vi "Update Step Descriptions.vi"(7 "Action":T1, 10 "Mouse Interaction Tag":string, 11 "UI Data in":refnum<class "Settings UI.lvclass">) -> (3 "UI Data out":refnum<class "Settings UI.lvclass">)   [LabVIEW 2020, in "Output Sequencer.lvlib" / "Settings UI.lvclass"]
uses:
  Settings UI.lvclass
  Types/Settings UI Action.ctl
  Settings UI.lvclass/Settings UI.ctl
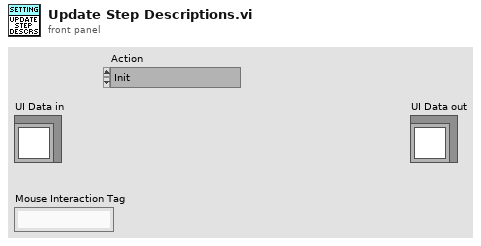
[diagram p1: front panel]
types:
  T1 = typedef "Output Sequencer.lvlib/Settings UI.lvclass/Settings UI Action.ctl" = enum16{"Init", "Timeout", "Tree Change", "Tree Mouse Down/Up", "Value Change", "Expand All", "Show Overview", "Collapse All", "Insert Above", "Insert Below", "Remove Step", "Move Up", "Move Down", "Drag Starting", "Drag Over", "Drop", "Drag Ended", "Import"}
  T2 = typedef "Output Sequencer.lvlib/Settings UI.lvclass/Step Settings.ctl" = cluster{"Description":string, "Precondition":string, "Duration":dbl, "Mode":string, "Delay Between Values":dbl, "Analog Values":string[], "Digital Values":string[], "Postcondition":string, "On True":string, "On False":string}
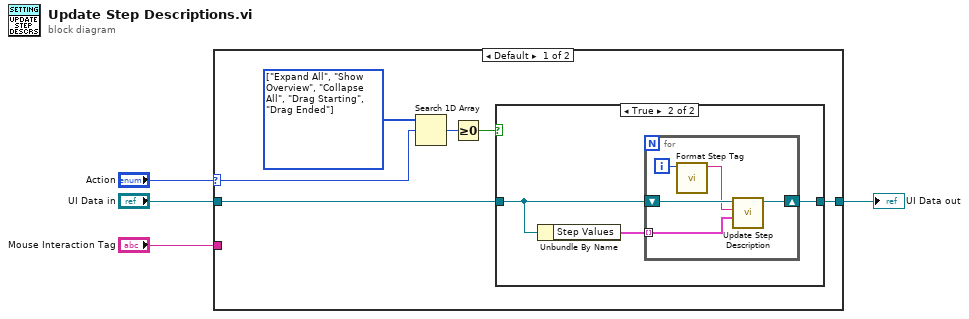
[diagram p0: block diagram]
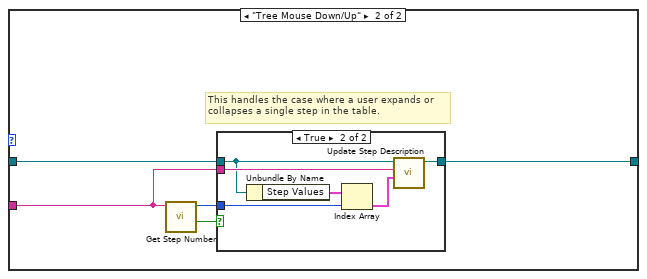
[diagram p3: hidden frame]
diagram:
  n1 = case shown="Default" "Action" {
    selector: "Action" -> [w9 _]
    tunnel: "UI Data in" -> [w7 w24]
    tunnel: "Mouse Interaction Tag" -> [_ w21]
    tunnel: [w5 w20] -> w1
    frame Default {
      w6 = T1[] [enum."Expand All", enum."Show Overview", enum."Collapse All", enum."Drag Starting", enum."Drag Ended"] items=["Init", "Timeout", "Tree Change", "Tree Mouse Down/Up", "Value Change", "Expand All", "Show Overview", "Collapse All", "Insert Above", "Insert Below", "Remove Step", "Move Up", "Move Down", "Drag Starting", "Drag Over", "Drop", "Drag Ended", "Import"]
      n2 = Search 1D Array(1D array=w6, element=w9) -> (index of element=w10:i32)  [unwired: 1 in]
      n3 = Greater Or Equal To 0?(x=w10) -> (x >= 0?=w8:bool)
      n4 = case shown="True" w8 {
        tunnel: w7 -> [w11 w13]
        tunnel: [w11 w12] -> w5
        frame False {
        }
        frame True {
          n5 = Unbundle By Name(w13) -> ("Step Values"=w14:T2[])
          n6 = for {
            tunnel: w14 -> [w19] mode=indexing
            shift-right: [w15] -> w12
            shift-left: w13 -> [w18]
            i -> [w17]
            n7 = call "Format Step Tag.vi"("Step Number"=w17) -> ("Tag"=w16:string)  [unwired: 10 in]
            n8 = call "Update Step Description.vi"("Step Settings"=w19, "Step tag"=w16, "UI Data in"=w18) -> ("UI Data out"=w15:refnum<class "Settings UI.lvclass">)  [unwired: 8 in]
          }
        }
      }
    }
    frame "Tree Mouse Down/Up" {
      # "This handles the case where a user expands or\ncollapses a single step in the table."
      n9 = call "Get Step Number.vi"("Tree Tag"=w21) -> ("Is Step tag?"=w22:bool, "Step Number"=w23:i32)  [unwired: 8 in, 1 out]
      n10 = case shown="True" w22 {
        tunnel: w24 -> [w25 w27]
        tunnel: w23 -> [_ w30]
        tunnel: w21 -> [_ w29]
        tunnel: [w25 w26] -> w20
        frame False {
        }
        frame True {
          n11 = Unbundle By Name(w27) -> ("Step Values"=w31:T2[])
          n12 = Index Array(array=w31, index=w30) -> (element=w28:T2)
          n13 = call "Update Step Description.vi"("Step Settings"=w28, "Step tag"=w29, "UI Data in"=w27) -> ("UI Data out"=w26:refnum<class "Settings UI.lvclass">)  [unwired: 8 in]
        }
      }
    }
  }
  "UI Data out" <- w1
